vi "Node Type.vi"(8 "error in (no error)":errorcluster, 11 "JSON Tree In":variant) -> (0 "error out":errorcluster, 2 "Value":variant, 3 "JSON Tree Passthrough":variant, 5 "JSON Compatible Type":T1=enum."Unknown", 7 "JSON Type":T2=enum."Unknown")   [LabVIEW 2013, in "i3-json.lvlib"]
doc: "Use this template to build a VI to use as a subVI."
uses:
  i3-json.lvlib
  JSON Types/JSON Type.ctl
  JSON Types/JSON Compatible Type.ctl
  JSON Types/JSON Variant Attribute.ctl
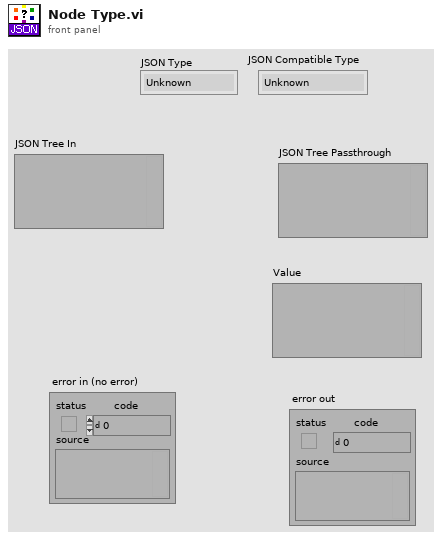
[diagram p1: front panel]
types:
  T1 = typedef "i3-json.lvlib/JSON Compatible Type.ctl" = enum16{"1D Double Array", "1D String Array", "1D Boolean Array", "Unknown"}
  T2 = typedef "i3-json.lvlib/JSON Type.ctl" = enum8{"JSON Compatible", "JSON Array", "JSON Object", "JSON Null", "Double", "String", "Boolean", "Unknown", "Data JSON string"}
  T3 = typedef "i3-json.lvlib/JSON Variant Attribute.ctl" = string
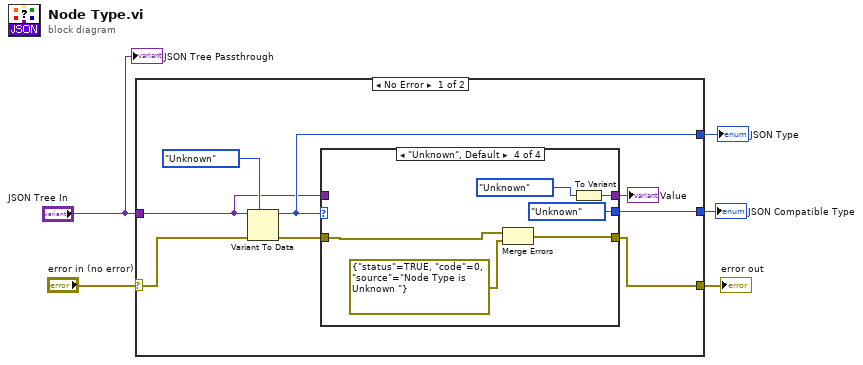
[diagram p0: block diagram]
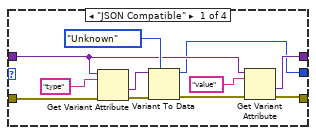
[diagram p2: hidden frame]
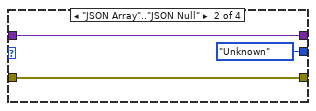
[diagram p3: hidden frame]
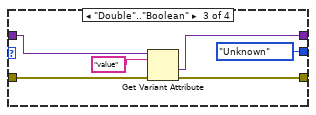
[diagram p4: hidden frame]
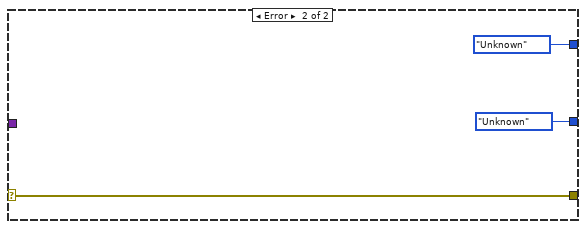
[diagram p5: hidden frame]
diagram:
  n1 = case shown="No Error" "error in (no error)" {
    selector: "error in (no error)" -> [w12 w42]
    tunnel: [w8 w42] -> w4
    tunnel: [w10 JSON_Compatible_Type."Unknown" ("JSON Compatible Type")] -> w3
    tunnel: [w9 JSON_Type."Unknown" ("JSON Type")] -> w2
    tunnel: "JSON Tree In" -> [w7 _]
    frame No Error {
      n2 = Variant To Data(error in=w12, type=JSON_Type."Unknown" ("JSON Type"), Variant=w7) -> (data=w9:T2, error out=w11:errorcluster)
      n3 = case shown="\"Unknown\", Default" w9 {
        tunnel: w7 -> [w16 w25 w32 _]
        tunnel: w11 -> [w24 w26 w30 w36]
        tunnel: [w14 JSON_Compatible_Type."Unknown" ("JSON Compatible Type") JSON_Compatible_Type."Unknown" ("JSON Compatible Type") JSON_Compatible_Type."Unknown" ("JSON Compatible Type")] -> w10
        tunnel: [w18 w26 w29 w34] -> w8
        tunnel: [w15 w25 w28 w39] -> w6
        frame "JSON Compatible" {
          n4 = Get Variant Attribute(Variant=w16, name=T3 "type" ("JSON Variant Attribute"), error in=w24) -> (value=w21:variant, error out=w22:errorcluster)  [unwired: 1 in, 2 out]
          n5 = Variant To Data(error in=w22, type=JSON_Compatible_Type."Unknown" ("JSON Compatible Type"), Variant=w21) -> (data=w14:T1, error out=w19:errorcluster)
          n6 = Get Variant Attribute(Variant=w16, name=T3 "value" ("JSON Variant Attribute"), error in=w19) -> (value=w15:variant, error out=w18:errorcluster)  [unwired: 1 in, 2 out]
        }
        frame "JSON Array".."JSON Null" {
        }
        frame "Double".."Boolean" {
          n7 = Get Variant Attribute(Variant=w32, name=T3 "value" ("JSON Variant Attribute"), error in=w30) -> (value=w28:variant, error out=w29:errorcluster)  [unwired: 1 in, 2 out]
        }
        frame "Unknown", Default {
          n8 = Merge Errors(w36, errorcluster {"status"=TRUE, "code"=0, "source"="Node Type is Unknown "} ("error out")) -> (w34:errorcluster)
          n9 = To Variant(anything=JSON_Type."Unknown" ("JSON Type")) -> (Variant=w39:variant)
        }
      }
      "Value" <- w6
    }
    frame Error {
    }
  }
  "error out" <- w4
  "JSON Compatible Type" <- w3
  "JSON Type" <- w2
  "JSON Tree Passthrough" <- "JSON Tree In"
